vi "Authentication.vi"(8 "error in (no error)":errorcluster, 11 "Hello in":refnum<class "Hello.lvclass">) -> (0 "error out":errorcluster, 2 "Authentication":T1, 3 "Hello out":refnum<class "Hello.lvclass">)   [LabVIEW 2022 SP3, in "obs-websocket-lv.lvlib" / "Hello.lvclass"]
uses:
  Hello.lvclass
  Hello.lvclass/Hello.ctl
  Authentication.ctl
  obs-websocket-lv.lvlib
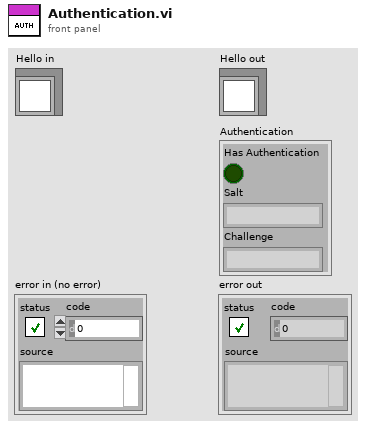
[diagram p1: front panel]
types:
  T1 = typedef "obs-websocket-lv.lvlib/Authentication.ctl" = cluster{"Has Authentication":bool, "Salt":string, "Challenge":string}
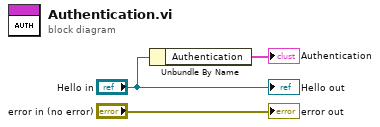
[diagram p0: block diagram]
diagram:
  n1 = Unbundle By Name("Hello in") -> ("Authentication"=→"Authentication":T1)
  "error out" <- "error in (no error)"
  "Hello out" <- "Hello in"
